vi "CRYData View Legend Item Delete.vi"(10 "RowNumber":i32=1, 11 "Legend MultiListbox In":refnum<vi>) -> (3 "Legend MultiListbox Out":refnum<vi>)   [LabVIEW 2013]
uses:
  <vilib>/Utility/miscctls.llb/LVRowAndColumnTypeDef.ctl
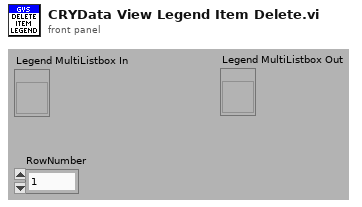
[diagram p1: front panel]
types:
  T1 = typedef "LVRowAndColumnTypeDef.ctl" = cluster{"Row":i32, "Column":i32}
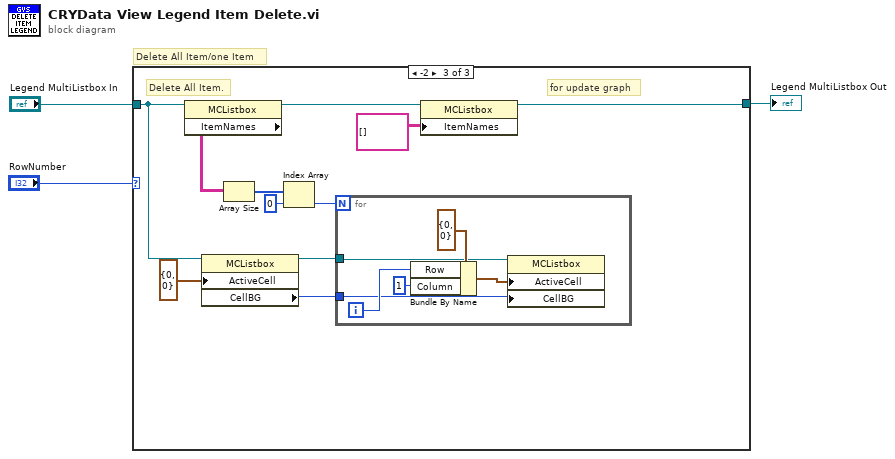
[diagram p0: block diagram]
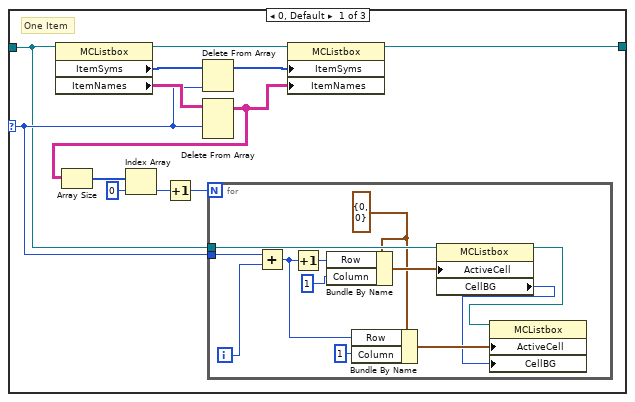
[diagram p2: hidden frame]
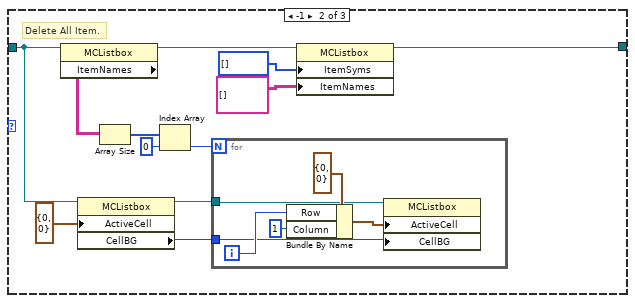
[diagram p3: hidden frame]
diagram:
  # "Delete All Item/one Item"
  n1 = case shown="-2" "RowNumber" {
    selector: "RowNumber" -> [w8 _ _]
    tunnel: "Legend MultiListbox In" -> [w7 w28 w46]
    tunnel: [w4 w29 w47] -> w1
    frame 0, Default {
      # "One Item"
      n2 = property on="Property Node" class="MCListbox"(reference=w7) -> (reference out=w13:refnum<vi>, "ItemSyms"=w14:i32[], "ItemNames"=w12:string[][])  [unwired: 1 in, 1 out]
      n3 = Delete From Array(array=w14, index=w8) -> (array with subset deleted=w15:i32[])  [unwired: 1 in, 1 out]
      n4 = Delete From Array(array=w12, index (row)=w8) -> (array with subset deleted=w11:string[][])  [unwired: 2 in, 1 out]
      n5 = Array Size(array=w11) -> (size(s)=w10:i32[])
      n6 = Index Array(array=w10, index=0) -> (element=w6:i32)
      n7 = Increment(x=w6) -> (x+1=w5:i32)
      n8 = for {
        N: w5 -> [_]
        tunnel: w8 -> [w27]
        tunnel: w7 -> [w22]
        i -> [w26]
        w20 = T1 {"Row"=0, "Column"=0} ("Active Cell:Active Cell")
        n9 = Add(x=w27, y=w26) -> (x+y=w17:i32)
        n10 = Increment(x=w17) -> (x+1=w19:i32)
        n11 = Bundle By Name(cluster=w20, "Row"=w19, "Column"=1) -> (w21:T1)
        n12 = Bundle By Name(cluster=w20, "Row"=w17, "Column"=1) -> (w24:T1)
        n13 = property on="Property Node" class="MCListbox"(reference=w22, "ActiveCell"=w21) -> (reference out=w23:refnum<vi>, "CellBG"=w16:u32)  [unwired: 1 in, 1 out]
        n14 = property on="Property Node" class="MCListbox"(reference=w23, "ActiveCell"=w24, "CellBG"=w16) -> ()  [unwired: 1 in, 2 out]
      }
      n15 = property on="Property Node" class="MCListbox"(reference=w13, "ItemSyms"=w15, "ItemNames"=w11) -> (reference out=w4:refnum<vi>)  [unwired: 1 in, 1 out]
    }
    frame -1 {
      # "Delete All Item."
      n16 = property on="Property Node" class="MCListbox"(reference=w28) -> (reference out=w31:refnum<vi>, "ItemNames"=w34:string[][])  [unwired: 1 in, 1 out]
      n17 = property on="Property Node" class="MCListbox"(reference=w28, "ActiveCell"=T1 {"Row"=0, "Column"=0} ("Active Cell:Active Cell")) -> (reference out=w30:refnum<vi>, "CellBG"=w32:u32)  [unwired: 1 in, 1 out]
      n18 = Array Size(array=w34) -> (size(s)=w37:i32[])
      n19 = Index Array(array=w37, index=0) -> (element=w35:i32)
      n20 = for {
        N: w35 -> [_]
        tunnel: w32 -> [w41]
        tunnel: w30 -> [w40]
        i -> [w42]
        n21 = Bundle By Name(cluster=T1 {"Row"=0, "Column"=0} ("Active Cell:Active Cell"), "Row"=w42, "Column"=1) -> (w44:T1)
        n22 = property on="Property Node" class="MCListbox"(reference=w40, "ActiveCell"=w44, "CellBG"=w41) -> ()  [unwired: 1 in, 2 out]
      }
      n23 = property on="Property Node" class="MCListbox"(reference=w31, "ItemSyms"=i32[] [] ("Item Symbols"), "ItemNames"=string[][] [] ("Item Names")) -> (reference out=w29:refnum<vi>)  [unwired: 1 in, 1 out]
    }
    frame -2 {
      # "for update graph"
      # "Delete All Item."
      n24 = property on="Property Node" class="MCListbox"(reference=w46) -> (reference out=w49:refnum<vi>, "ItemNames"=w52:string[][])  [unwired: 1 in, 1 out]
      n25 = property on="Property Node" class="MCListbox"(reference=w46, "ActiveCell"=T1 {"Row"=0, "Column"=0} ("Active Cell:Active Cell")) -> (reference out=w48:refnum<vi>, "CellBG"=w50:u32)  [unwired: 1 in, 1 out]
      n26 = Array Size(array=w52) -> (size(s)=w55:i32[])
      n27 = Index Array(array=w55, index=0) -> (element=w53:i32)
      n28 = for {
        N: w53 -> [_]
        tunnel: w50 -> [w58]
        tunnel: w48 -> [w57]
        i -> [w59]
        n29 = Bundle By Name(cluster=T1 {"Row"=0, "Column"=0} ("Active Cell:Active Cell"), "Row"=w59, "Column"=1) -> (w61:T1)
        n30 = property on="Property Node" class="MCListbox"(reference=w57, "ActiveCell"=w61, "CellBG"=w58) -> ()  [unwired: 1 in, 2 out]
      }
      n31 = property on="Property Node" class="MCListbox"(reference=w49, "ItemNames"=string[][] [] ("Item Names")) -> (reference out=w47:refnum<vi>)  [unwired: 1 in, 1 out]
    }
  }
  "Legend MultiListbox Out" <- w1
